vi "20190424 Subvi AO trigger.vi"(9 "Delay_ticks":u32, 11 "Trigger":bool) -> (1 "IteratorDirection":bool, 3 "Stop":bool)   [LabVIEW 2017]
uses:
  GV trigger external AODO.vi
  GV Nframes.vi
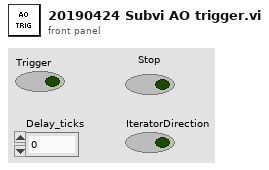
[diagram p1: front panel]
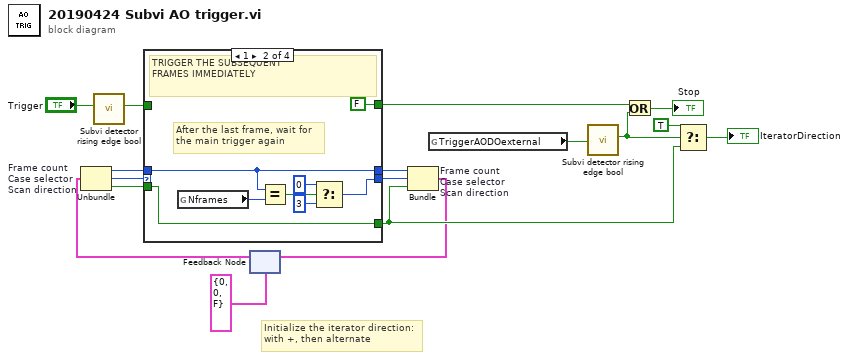
[diagram p0: block diagram]
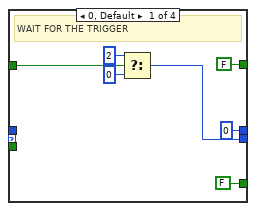
[diagram p2: hidden frame]
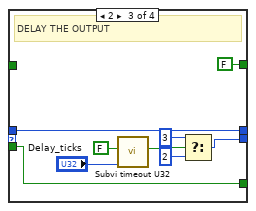
[diagram p3: hidden frame]
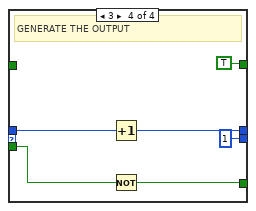
[diagram p4: hidden frame]
diagram:
  # "Initialize the iterator direction:\nwith +, then alternate"
  n1 = call "Subvi detector rising edge bool.vi"("Input"="Trigger") -> ("Output"=w8:bool)  [unwired: 10 in]
  n2 = feedback #1(cluster{i16, "f":u8, bool} {0, "f"=0, FALSE}) -> (w6:cluster{i16, "f":u8, bool})
  n3 = Unbundle "Frame count\nCase selector\nScan direction"(w6) -> (w5:i16, "f"=w3:u8, w4:bool)
  n4 = case shown="1" w3 {
    tunnel: [w24 w30 w39 u8 1 ("f")] -> w15
    tunnel: [FALSE FALSE FALSE TRUE] -> w11
    tunnel: [FALSE w26 w37 w45] -> w12
    tunnel: w8 -> [w20 _ _ _]
    tunnel: [i16 0 w25 w33 w42] -> w1
    tunnel: w4 -> [_ w26 w37 w44]
    tunnel: w5 -> [_ w25 w33 w43]
    frame 0, Default {
      # "WAIT FOR THE TRIGGER"
      n5 = Select(t=u8 2, s=w20, f=u8 0) -> (s? t:f=w24:u8)
    }
    frame 1 {
      # "After the last frame, wait for\nthe main trigger again"
      # "TRIGGER THE SUBSEQUENT\nFRAMES IMMEDIATELY"
      n6 = global read "GV Nframes.vi" "Nframes"() -> (w27:i16)
      n7 = Equal?(x=w25, y=w27) -> (x = y?=w28:bool)
      n8 = Select(t=u8 0, s=w28, f=u8 3) -> (s? t:f=w30:u8)
    }
    frame 2 {
      # "DELAY THE OUTPUT"
      n9 = call "Subvi timeout U32.vi"("Timeout_tick"="Delay_ticks", "Input"=FALSE) -> ("Timeout"=w34:bool)  [unwired: 9 in]
      n10 = Select(t=u8 3, s=w34, f=u8 2) -> (s? t:f=w39:u8)
    }
    frame 3 {
      # "GENERATE THE OUTPUT"
      n11 = Increment(x=w43) -> (x+1=w42:i16)
      n12 = Not(x=w44) -> (.not. x?=w45:bool)
    }
  }
  n13 = Bundle "Frame count\nCase selector\nScan direction"(w1, "f"=w15, w12) -> (w7:cluster{i16, "f":u8, bool})  [unwired: 1 in]
  n14 = feedback-in #1(w7) -> ()
  n15 = global read "GV trigger external AODO.vi" "TriggerAODOexternal"() -> (w17:bool)
  n16 = call "Subvi detector rising edge bool.vi"("Input"=w17) -> ("Output"=w10:bool)  [unwired: 10 in]
  n17 = Or(x=w11, y=w10) -> (x .or. y?=→"Stop":bool)
  n18 = Select(t=TRUE, s=w10, f=w12) -> (s? t:f=→"IteratorDirection":bool)
